vi "initalize gating(SubVI).vi"(0 "簇":T1={"initialize"=enum."SR830", "6221"={"6221 Resource"="GPIB0::24::INSTR", "Delta status"=FALSE, "电流"=0.0}, "SR830+6221"={"source"=0, "阻抗"=0.0, "量程入 4"=0, "量程入 3"=0, "量程入 2"=0, "量程入 1"=0, "SR830 2"=FALSE, "SR830 3"=FALSE, "SR830 4"=FALSE, "SR830 1"=FALSE, "VISA 1"="", "VISA 2"="", "VISA 3"="", "VISA 4"="", "Reserve 1"=0, "Reserve 2"=-1, "Reserve 3"=-1, "Reserve 4"=-1, "量程"=enum."量程每次测量会判定"}, "2400"={"2400"=FALSE, "VISA"=""}, "ch"={"ch"=[], "current"=[], "change?"=[], "holding current\nwhen change ch?"=FALSE}, "Instrument"={"335 Resource"="GPIB0::24::INSTR", "Input (0:A)"=0, "Instrument Type"=enum."SVSM", "quantum design"=refnum, "Heater Output (1:1)"=1, "semaphore"=refnum, "TCP master instance"=refnum, "335 Status"=refnum, "M24C Resource"="GPIB0::24::INSTR", "4G supply"="GPIB0::24::INSTR", "Temp Status 24C"=refnum, "Temp"=refnum, "9T信号"=refnum, "limit"={"Field limit"=0.0, "Field rate limit"=0.0, "Temp limit"=0.0, "Temp low limit"=0.0, "Temp rate limit "=0.0}, "4g supply status"=refnum}, "Aborting"=refnum, "数据文件"=refnum, "warning"=refnum} {"Instrument"."Input (0:A)" items=["A", "B"]; "Instrument"."Heater Output (1:1)" items=["1"=1, "2"=2]; "SR830+6221"."Reserve 4" items=["Auto Reserve"=-1, "High Reserve"=0, "Normal"=1, "Low Noise"=2]; "SR830+6221"."Reserve 3" items=["Auto Reserve"=-1, "High Reserve"=0, "Normal"=1, "Low Noise"=2]; "SR830+6221"."Reserve 2" items=["Auto Reserve"=-1, "High Reserve"=0, "Normal"=1, "Low Noise"=2]; "SR830+6221"."Reserve 1" items=["量程每次测量会判定", "量程不变为设定值"]; "SR830+6221"."source" items=["SR830 1", "SR830 2", "SR830 3", "SR830 4"]}, 2 "字符串":string) -> (7 "输出簇":T1={"initialize"=enum."SR830", "6221"={"6221 Resource"="GPIB0::24::INSTR", "Delta status"=FALSE, "电流"=0.0}, "SR830+6221"={"source"=0, "阻抗"=0.0, "量程入 4"=0, "量程入 3"=0, "量程入 2"=0, "量程入 1"=0, "SR830 2"=FALSE, "SR830 3"=FALSE, "SR830 4"=FALSE, "SR830 1"=FALSE, "VISA 1"="", "VISA 2"="", "VISA 3"="", "VISA 4"="", "Reserve 1"=0, "Reserve 2"=-1, "Reserve 3"=-1, "Reserve 4"=-1, "量程"=enum."量程每次测量会判定"}, "2400"={"2400"=FALSE, "VISA"=""}, "ch"={"ch"=[], "current"=[], "change?"=[], "holding current\nwhen change ch?"=FALSE}, "Instrument"={"335 Resource"="GPIB0::24::INSTR", "Input (0:A)"=0, "Instrument Type"=enum."SVSM", "quantum design"=refnum, "Heater Output (1:1)"=1, "semaphore"=refnum, "TCP master instance"=refnum, "335 Status"=refnum, "M24C Resource"="GPIB0::24::INSTR", "4G supply"="GPIB0::24::INSTR", "Temp Status 24C"=refnum, "Temp"=refnum, "9T信号"=refnum, "limit"={"Field limit"=0.0, "Field rate limit"=0.0, "Temp limit"=0.0, "Temp low limit"=0.0, "Temp rate limit "=0.0}, "4g supply status"=refnum}, "Aborting"=refnum, "数据文件"=refnum, "warning"=refnum} {"Instrument"."Input (0:A)" items=["A", "B"]; "Instrument"."Heater Output (1:1)" items=["1"=1, "2"=2]; "SR830+6221"."Reserve 4" items=["Auto Reserve"=-1, "High Reserve"=0, "Normal"=1, "Low Noise"=2]; "SR830+6221"."Reserve 3" items=["Auto Reserve"=-1, "High Reserve"=0, "Normal"=1, "Low Noise"=2]; "SR830+6221"."Reserve 2" items=["Auto Reserve"=-1, "High Reserve"=0, "Normal"=1, "Low Noise"=2]; "SR830+6221"."Reserve 1" items=["量程每次测量会判定", "量程不变为设定值"]; "SR830+6221"."source" items=["SR830 1", "SR830 2", "SR830 3", "SR830 4"]})   [LabVIEW 2019, in "initialize.lvlib"]
uses:
  initialize.lvlib
  config.ctl
  <vilib>/NI/Modbus Library/API/Master/Modbus Master.lvclass
  initialize.ctl
  Instrument.ctl
  Instrument Type.ctl
  lib/QDInstrument.dll
  335 state.ctl
  limit.ctl
  9T mag field stauts.ctl
  warning.ctl
  lib/Keithley 24XX/Keithley 24XX.lvlib
  Get value.lvlib
panel:
  in  "Compliance  Level (A)":dbl=0.0001
  in  "2400 resource name":refnum<visa-resource-name>
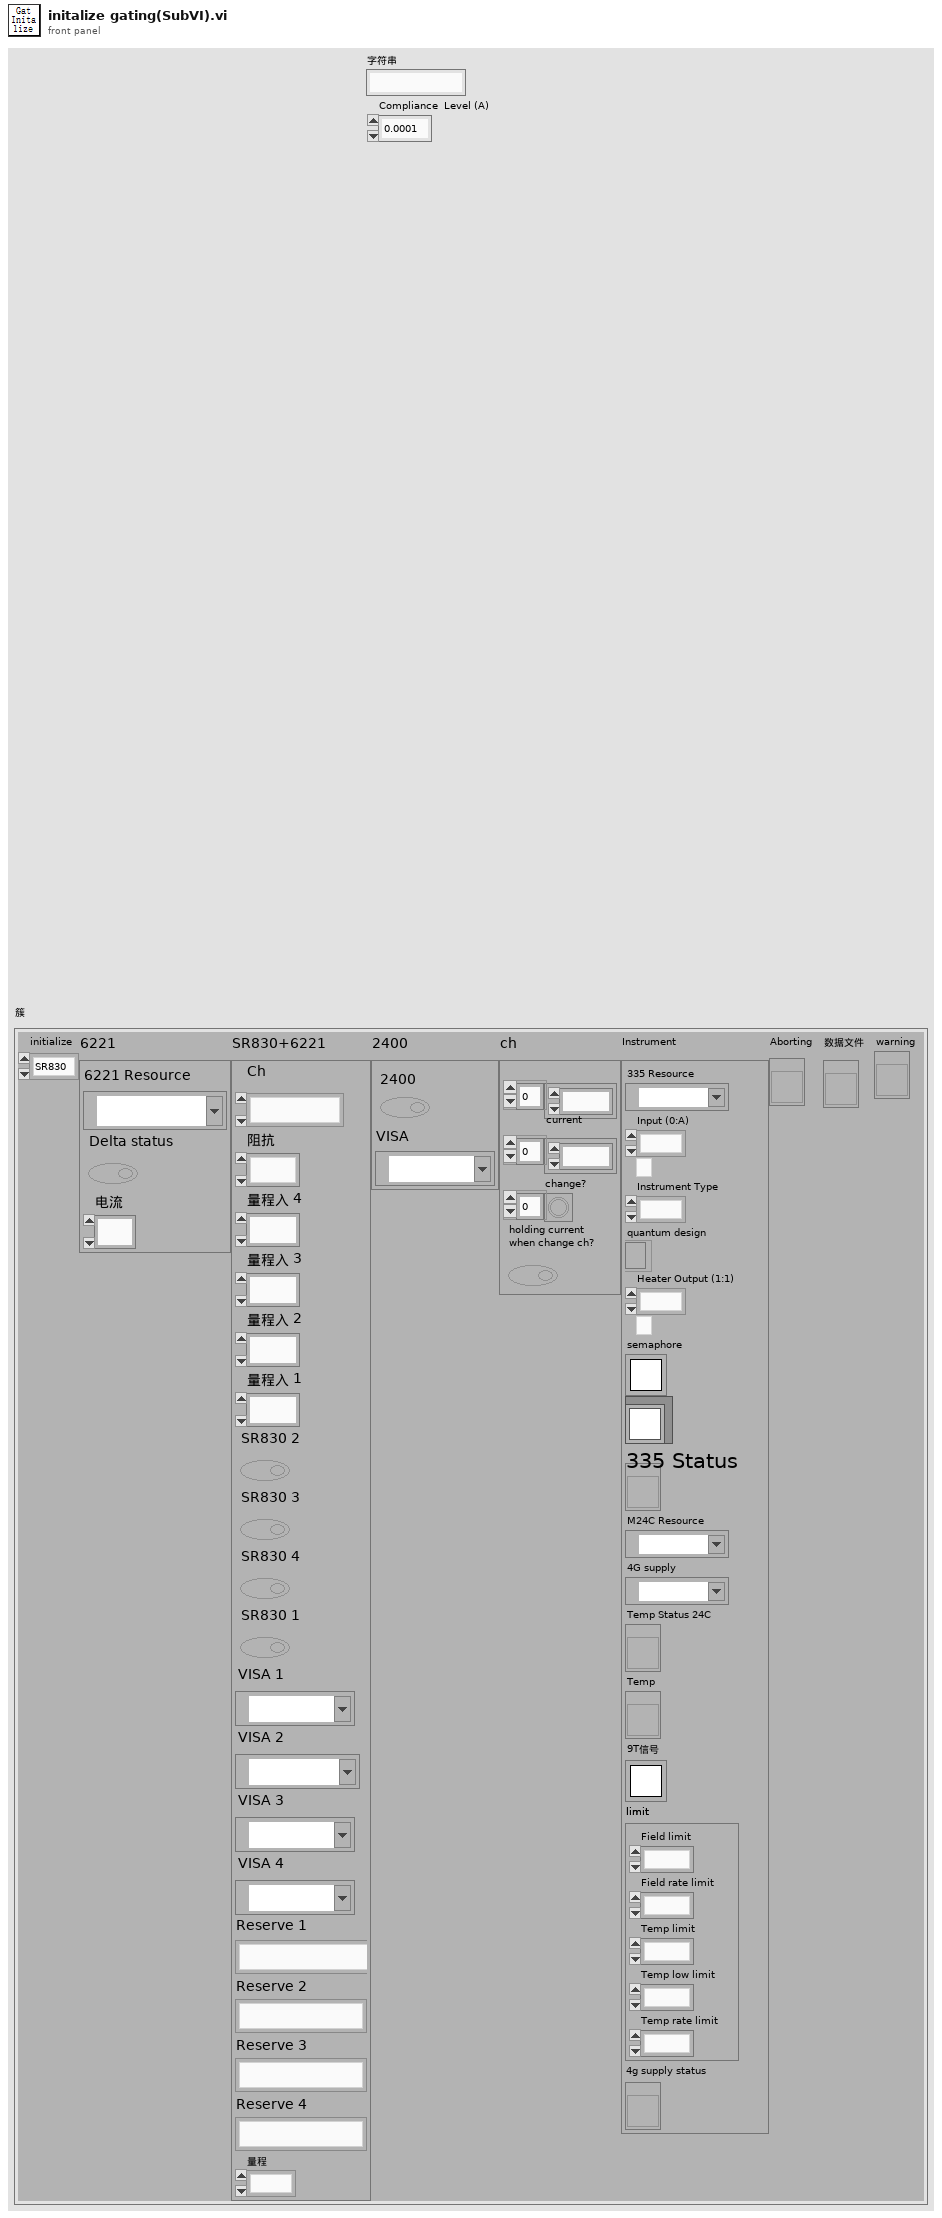
[diagram p1: front panel]
types:
  T1 = typedef "config.ctl" = cluster{"initialize":T2, "6221":cluster{"6221 Resource":refnum<visa-resource-name>, "Delta status":bool, "电流":dbl}, "SR830+6221":cluster{"source":u16, "阻抗":dbl, "量程入 4":i32, "量程入 3":i32, "量程入 2":i32, "量程入 1":i32, "SR830 2":bool, "SR830 3":bool, "SR830 4":bool, "SR830 1":bool, "VISA 1":refnum<visa-resource-name>, "VISA 2":refnum<visa-resource-name>, "VISA 3":refnum<visa-resource-name>, "VISA 4":refnum<visa-resource-name>, "Reserve 1":i16, "Reserve 2":i16, "Reserve 3":i16, "Reserve 4":i16, "量程":enum16{"量程每次测量会判定", "量程不变为设定值"}}, "2400":cluster{"2400":bool, "VISA":refnum<visa-resource-name>}, "ch":cluster{"ch":i32[], "current":dbl[], "change?":bool[], "holding current\nwhen change ch?":bool}, "Instrument":T3, "Aborting":refnum<vi>, "数据文件":refnum<vi>, "warning":refnum<vi>}
  T2 = typedef "initialize.ctl" = enum16{"SR830", "keithley6221-SR830", "Delta", "Delta-tunnelling", "keithley6221-2182-DC"}
  T3 = typedef "Instrument.ctl" = cluster{"335 Resource":refnum<visa-resource-name>, "Input (0:A)":u16, "Instrument Type":T4, "quantum design":refnum<k24>, "Heater Output (1:1)":u16, "semaphore":T5, "TCP master instance":refnum<class "Modbus Master.lvclass">, "335 Status":refnum<vi>, "M24C Resource":refnum<visa-resource-name>, "4G supply":refnum<visa-resource-name>, "Temp Status 24C":refnum<vi>, "Temp":refnum<vi>, "9T信号":T5, "limit":T6, "4g supply status":refnum<vi>}
  T4 = typedef "Instrument Type.ctl" = enum16{"PPMS", "VersaLab", "DynaCool", "SVSM", "PPMS-Rotate", "Lakeshore335", "9T mag"}
  T5 = typedef "Semaphore RefNum" = refnum<k1>
  T6 = typedef "limit.ctl" = cluster{"Field limit":dbl, "Field rate limit":dbl, "Temp limit":dbl, "Temp low limit":dbl, "Temp rate limit ":dbl}
  T7 = typedef "Keithley 622x.lvlib/KE622x -- On Off Control.ctl" = enum16{"Off", "On"}
  T8 = cluster{"Baud Rate":u32, "Parity":u16, "Data Bits":u16, "Stop Bits":u16, "Flow Control":u16}
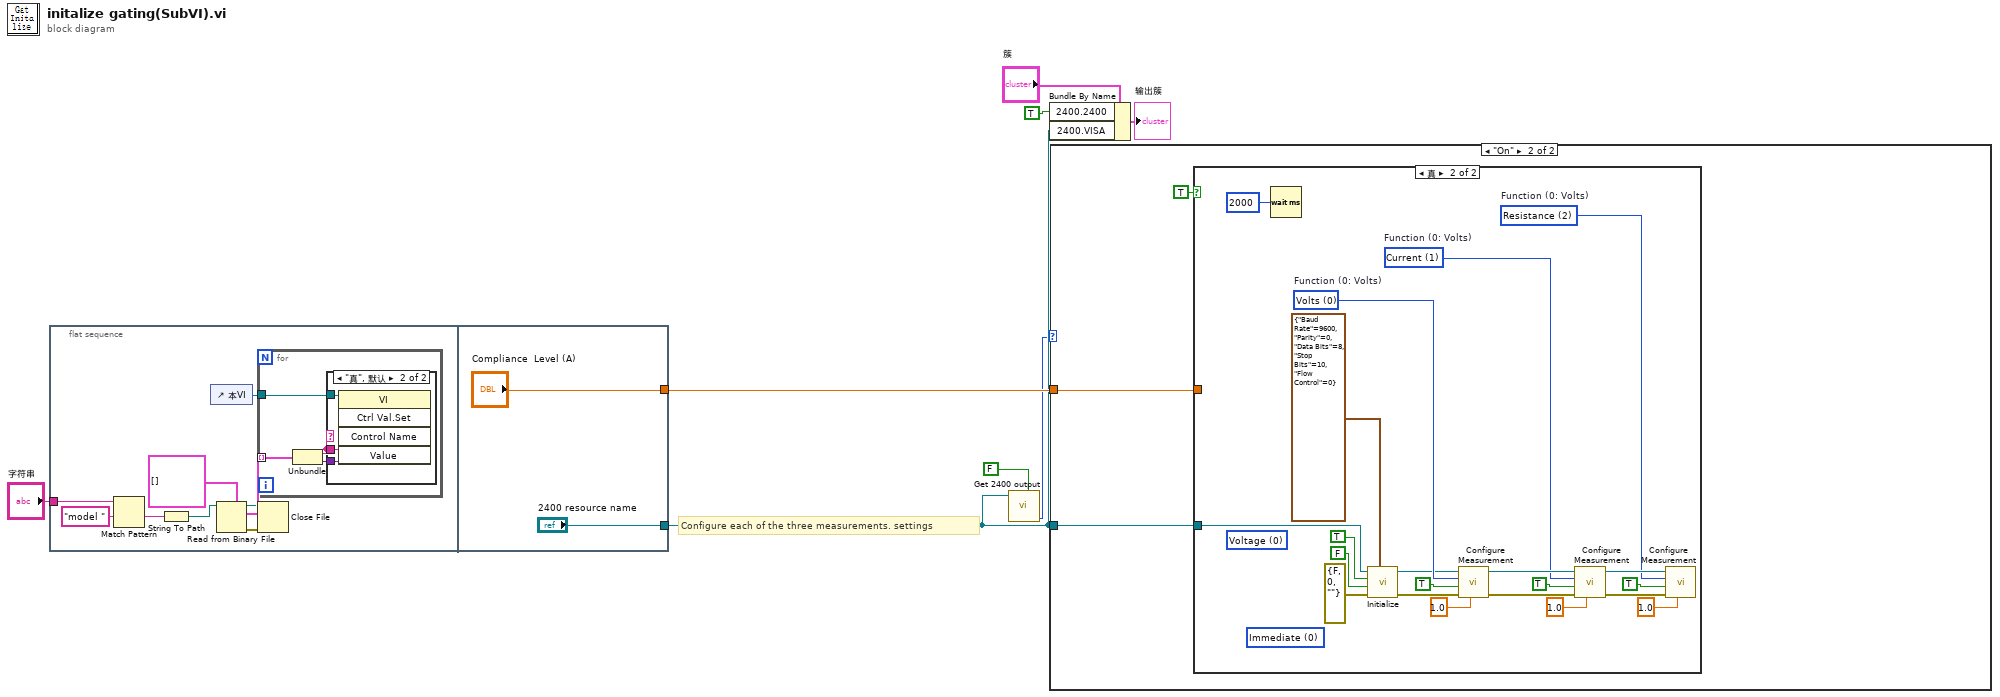
[diagram p0: block diagram]
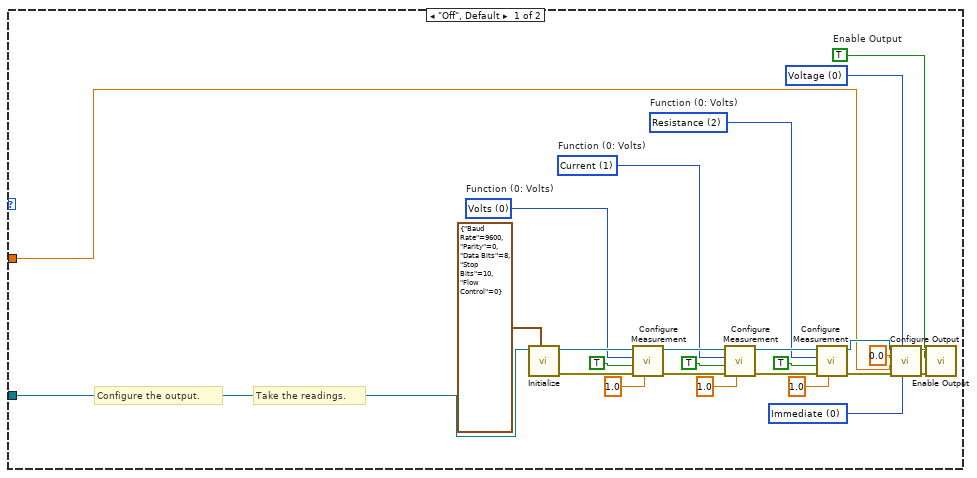
[diagram p2: hidden frame]
diagram:
  # "Configure each of the three measurements. settings"
  n1 = flat-sequence {
    tunnel: "字符串" -> [w17]
    tunnel: ["Compliance  Level (A)"] -> w7
    tunnel: ["2400 resource name"] -> w5
    frame #0 {
      n2 = Match Pattern(string=w17, regular expression="model " ("正则表达式")) -> (after substring=w16:string)  [unwired: 1 in, 3 out]
      n3 = String To Path(string=w16) -> (path=w13:path)
      n4 = control-ref of="本VI"() -> (w14:refnum<vi>)
      n5 = Read from Binary File(5:cluster{"Name":string, "Variant Data":variant}[] [] ("控件值:获取全部"), 11:w13) -> (0:w9:errorcluster, 2:w11:cluster{"Name":string, "Variant Data":variant}[], 3:w10:refnum<file>)  [unwired: 4 in, 1 out]
      n6 = for {
        tunnel: w11 -> [w21] mode=indexing
        tunnel: w14 -> [w20]
        n7 = Unbundle(w21) -> ("Name"=w18:string, "Variant Data"=w19:variant)
        n8 = case shown="\"真\", 默认" w18 {
          tunnel: w20 -> [_ w24]
          tunnel: w18 -> [_ w23]
          tunnel: w19 -> [_ w22]
          frame "cancel", "load", "model", "ok" {
          }
          frame "真", Default {
            n9 = invoke class="VI" method="Ctrl Val.Set"(reference=w24, "Control Name"=w23, "Value"=w22) -> ()  [unwired: 2 in, 5 out]
          }
        }
      }
      n10 = Close File(refnum=w10, error in=w9) -> ()  [unwired: 2 out]
    }
    frame #1 {
    }
  }
  n11 = call "Get 2400 output.vi"("Check For SCPI Errors? (T)"=FALSE, "Resource In"=w5) -> ("Output State"=w4:T7)  [unwired: 8 in, 1 out]
  n12 = Bundle By Name(cluster="簇", "2400.2400"=TRUE, "2400.VISA"=w5) -> (→"输出簇":T1)
  n13 = case shown="\"On\"" w4 {
    tunnel: w7 -> [w29 w53]
    tunnel: w5 -> [w28 w55]
    frame "Off", Default {
      w27 = u16 0 items=["Immediate", "Triggered"] ("Output Type  (0: Immediate)")
      w30 = u16 0 items=["Voltage", "Current"] ("Source Mode  (0: Voltage)")
      w33 = TRUE  # Enable Output
      w43 = u16 2 items=["Volts", "Current", "Resistance"]  # Function (0: Volts)
      w44 = u16 1 items=["Volts", "Current", "Resistance"]  # Function (0: Volts)
      w45 = u16 0 items=["Volts", "Current", "Resistance"]  # Function (0: Volts)
      # "Take the readings."
      # "Configure the output."
      n14 = call "Initialize.vi"("Serial Configuration"=T8 {"Baud Rate"=9600, "Parity"=0, "Data Bits"=8, "Stop Bits"=10, "Flow Control"=0}, "VISA resource name"=w28) -> ("error out"=w50:errorcluster, "VISA resource name out"=w51:refnum<visa-resource-name>)  [unwired: 8 in]
      n15 = call "Configure Measurement.vi"("Manual Range (1.0)"=1.0 ("Voltage Manual Range (1.0)"), "error in (no error)"=w50, "Enable Auto Range (T:Enable)"=TRUE ("Enable Voltage Auto Range (T:Enable)"), "Function (0: Volts)"=w45, "VISA resource name"=w51) -> ("error out"=w48:errorcluster, "VISA resource name out"=w49:refnum<visa-resource-name>)  [unwired: 5 in]
      n16 = call "Configure Measurement.vi"("Manual Range (1.0)"=1.0 ("Current Manual Range (1.0)"), "error in (no error)"=w48, "Enable Auto Range (T:Enable)"=TRUE ("Enable Current Auto Range (T:Enable)"), "Function (0: Volts)"=w44, "VISA resource name"=w49) -> ("error out"=w47:errorcluster, "VISA resource name out"=w46:refnum<visa-resource-name>)  [unwired: 5 in]
      n17 = call "Configure Measurement.vi"("Manual Range (1.0)"=1.0 ("Resistance Manual Range (1.0)"), "error in (no error)"=w47, "Enable Auto Range (T:Enable)"=TRUE ("Enable Resistance Auto Range (T:Enable)"), "Function (0: Volts)"=w43, "VISA resource name"=w46) -> ("error out"=w32:errorcluster, "VISA resource name out"=w31:refnum<visa-resource-name>)  [unwired: 5 in]
      n18 = call "Configure Output.vi"("Output Type  (0: Immediate)"=w27, "Source Mode  (0: Voltage)"=w30, "error in (no error)"=w32, "Compliance  Level (0.1)"=w29, "Output Level (0)"=0.0, "VISA resource name"=w31) -> ("error out"=w34:errorcluster, "VISA resource name out"=w35:refnum<visa-resource-name>)  [unwired: 4 in]
      n19 = call "Enable Output.vi"("error in (no error)"=w34, "Enable Output (T: Enable)"=w33, "VISA resource name"=w35) -> ()  [unwired: 7 in, 2 out]
    }
    frame "On" {
      n20 = case shown="真" TRUE {
        tunnel: w55 -> [_ w64]
        tunnel: w53 -> [_ _]
        frame False {
        }
        frame True {
          (unwired) u16 0 items=["Immediate", "Triggered"] ("Output Type  (0: Immediate)")
          (unwired) u16 0 items=["Voltage", "Current"] ("Source Mode  (0: Voltage)")
          w70 = u16 2 items=["Volts", "Current", "Resistance"]  # Function (0: Volts)
          w71 = u16 1 items=["Volts", "Current", "Resistance"]  # Function (0: Volts)
          w72 = u16 0 items=["Volts", "Current", "Resistance"]  # Function (0: Volts)
          n21 = Wait (ms)(milliseconds to wait=u32 2000) -> ()  [unwired: 1 out]
          n22 = call "Initialize.vi"("Serial Configuration"=T8 {"Baud Rate"=9600, "Parity"=0, "Data Bits"=8, "Stop Bits"=10, "Flow Control"=0}, "error in (no error)"=errorcluster {"status"=FALSE, "code"=0, "source"=""}, "Reset (True)"=FALSE, "ID Query (True)"=TRUE, "VISA resource name"=w64) -> ("error out"=w58:errorcluster, "VISA resource name out"=w63:refnum<visa-resource-name>)  [unwired: 5 in]
          n23 = call "Configure Measurement.vi"("Manual Range (1.0)"=1.0 ("Voltage Manual Range (1.0)"), "error in (no error)"=w58, "Enable Auto Range (T:Enable)"=TRUE ("Enable Voltage Auto Range (T:Enable)"), "Function (0: Volts)"=w72, "VISA resource name"=w63) -> ("error out"=w75:errorcluster, "VISA resource name out"=w76:refnum<visa-resource-name>)  [unwired: 5 in]
          n24 = call "Configure Measurement.vi"("Manual Range (1.0)"=1.0 ("Current Manual Range (1.0)"), "error in (no error)"=w75, "Enable Auto Range (T:Enable)"=TRUE ("Enable Current Auto Range (T:Enable)"), "Function (0: Volts)"=w71, "VISA resource name"=w76) -> ("error out"=w74:errorcluster, "VISA resource name out"=w73:refnum<visa-resource-name>)  [unwired: 5 in]
          n25 = call "Configure Measurement.vi"("Manual Range (1.0)"=1.0 ("Resistance Manual Range (1.0)"), "error in (no error)"=w74, "Enable Auto Range (T:Enable)"=TRUE ("Enable Resistance Auto Range (T:Enable)"), "Function (0: Volts)"=w70, "VISA resource name"=w73) -> ()  [unwired: 5 in, 2 out]
        }
      }
    }
  }
